vi "VALVE_read_position.vi"(4 "Valve adress":string, 5 "error in":errorcluster, 8 "VISA valve":refnum<visa-resource-name>) -> (0 "error out":errorcluster, 3 "Valve position OUT":u8)   [LabVIEW 2015]
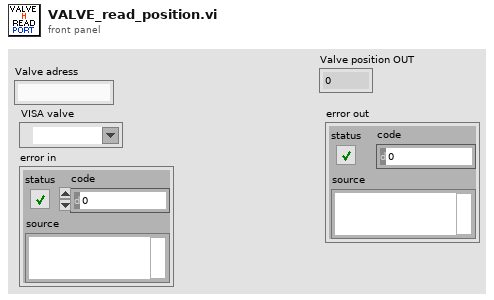
[diagram p1: front panel]
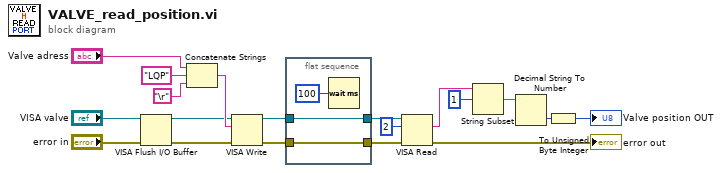
[diagram p0: block diagram]
diagram:
  n1 = VISA Flush I/O Buffer(VISA resource name="VISA valve", error in (no error)="error in") -> (VISA resource name out=w10:refnum<visa-resource-name>, error out=w11:errorcluster)  [unwired: 1 in]
  n2 = Concatenate Strings("Valve adress", "LQP" ("string"), "\r") -> (w13:string)
  n3 = VISA Write(VISA resource name=w10, write buffer=w13, error in (no error)=w11) -> (VISA resource name out=w8:refnum<visa-resource-name>, error out=w7:errorcluster)  [unwired: 1 out]
  n4 = flat-sequence {
    tunnel: w8 -> [w22]
    tunnel: [w22] -> w6
    tunnel: w7 -> [w21]
    tunnel: [w21] -> w5
    frame #0 {
      n5 = Wait (ms)(milliseconds to wait=u32 100) -> ()  [unwired: 1 out]
    }
  }
  n6 = VISA Read(VISA resource name=w6, byte count=u32 2, error in (no error)=w5) -> (read buffer=w15:string, error out=→"error out":errorcluster)  [unwired: 2 out]
  n7 = String Subset(string=w15, offset (0)=1) -> (substring=w17:string)  [unwired: 1 in]
  n8 = Decimal String To Number(string=w17) -> (number=w14:i32)  [unwired: 2 in, 1 out]
  n9 = To Unsigned Byte Integer(number=w14) -> (unsigned 8bit integer=→"Valve position OUT":u8)
